vi "module1.vi"(11 "controlRelays":u8) -> (3 "debugControlRelays":u8)   [LabVIEW 2021]
uses:
  <vilib>/rvi/eio/common/nirviEmuTemplateMethod_errors.vi
  <vilib>/eio/EIONode/EIONode.xnode
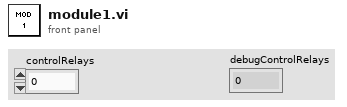
[diagram p1: front panel]
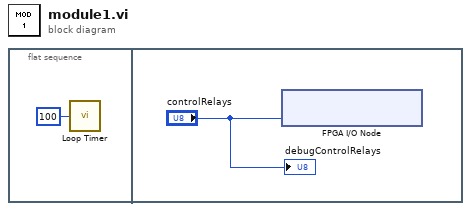
[diagram p0: block diagram]
diagram:
  n1 = flat-sequence {
    frame #0 {
      n2 = call "Loop Timer"("Count(mSec)"=u32 100) -> ()  [unwired: 1 out]
    }
    frame #1 {
      n3 = xnode "FPGA I/O Node"("Mod1/User LED3:0"="controlRelays") -> ()  [unwired: 1 in, 1 out]
      "debugControlRelays" <- "controlRelays"
    }
  }
